vi "Unpack Averaged Data.vi"(7 "Coordinate Space":T1 caption="Coord", 10 "Data":dbl[][](array[numeric]), 11 "Source Group":T2) -> (1 "Forces":dbl[](array[numeric]), 2 "Disp":dbl[](array[numeric]), 3 "Cmds":dbl[](array[numeric]))   [LabVIEW 2013]
uses:
  W:/NSEL OM/lib/Global Data/Names/Source Group Type.ctl
  Offsets Widget/Cartesian Or Actuator.ctl
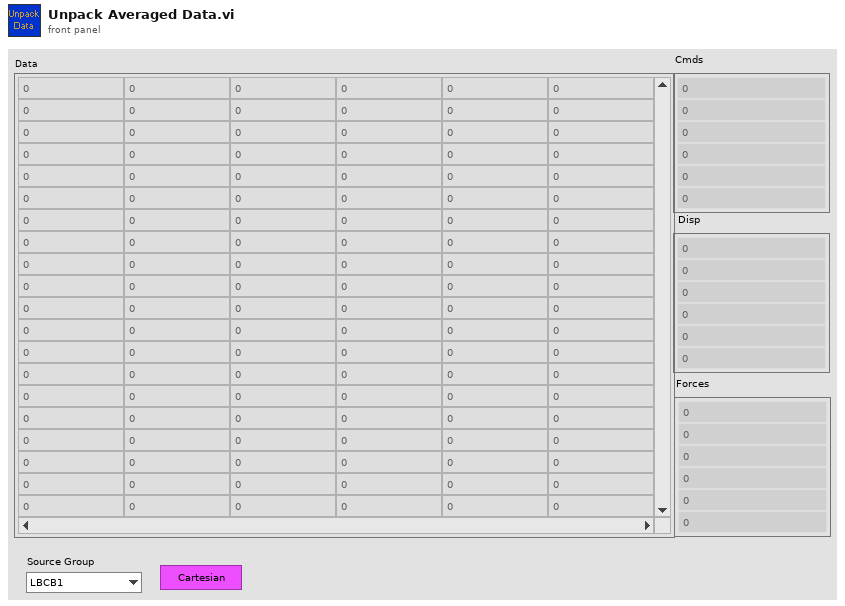
[diagram p1: front panel]
types:
  T1 = typedef "Cartesian Or Actuator.ctl" = bool
  T2 = typedef "Source Group Type.ctl" = enum16{"LBCB1", "LBCB2", "Consolidated", "External"}
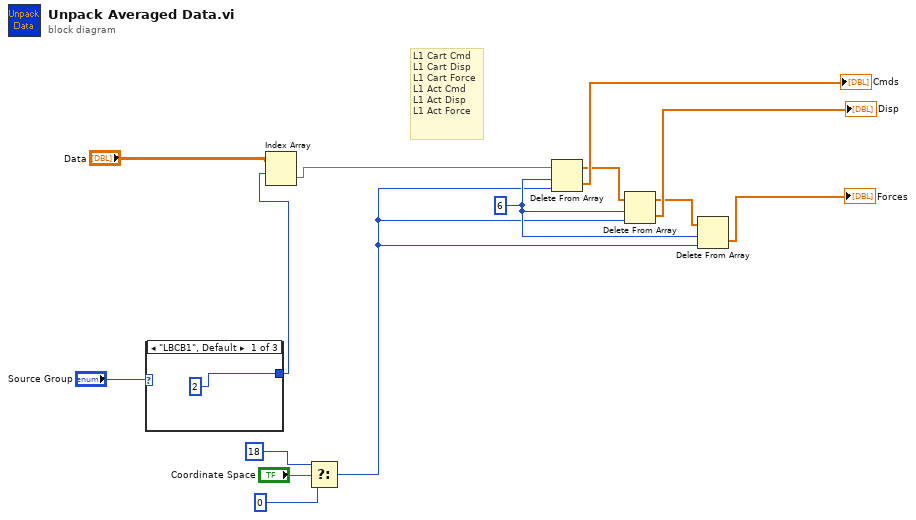
[diagram p0: block diagram]
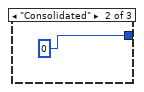
[diagram p2: hidden frame]
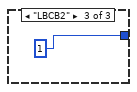
[diagram p3: hidden frame]
diagram:
  w2 = 6 ("length")
  # "L1 Cart Cmd\nL1 Cart Disp\nL1 Cart Force\nL1 Act Cmd\nL1 Act Disp\nL1 Act Force"
  n1 = case shown="\"LBCB1\", Default" "Source Group" {
    tunnel: [2 0 1] -> w12
    frame "LBCB1", Default {
    }
    frame "Consolidated" {
    }
    frame "LBCB2" {
    }
  }
  n2 = Index Array(array="Data", index (row)=w12) -> (element=w11:dbl[])  [unwired: 1 in]
  n3 = Select(t=18, s="Coordinate Space", f=0) -> (s? t:f=w1:i32)
  n4 = Delete From Array(array=w11, length=w2, index=w1) -> (deleted portion=→"Cmds":dbl[], array with subset deleted=w6:dbl[])
  n5 = Delete From Array(array=w6, length=w2, index=w1) -> (deleted portion=→"Disp":dbl[], array with subset deleted=w4:dbl[])
  n6 = Delete From Array(array=w4, length=w2, index=w1) -> (deleted portion=→"Forces":dbl[])  [unwired: 1 out]
